vi "Configure Digital Channel.vi"(5 "Threshold (1.4 V)":dbl=1.4, 6 "Channel Size (1: Medium)":i32(ring)=1 items=["Small", "Medium", "Large"], 7 "Channel Position (0)":dbl, 8 "error in (no error)":errorcluster, 9 "Enable Display (F: Disable)":bool, 10 "Channel Name (0: D0)":i32(ring) items=["D0", "D1", "D2", "D3", "D4", "D5", "D6", "D7", "D8", "D9", "D10", "D11", "D12", "D13", "D14", "D15"], 11 "VISA resource name":refnum<visa-resource-name>) -> (0 "error out":errorcluster, 3 "VISA resource name out":refnum<visa-resource-name>)   [LabVIEW 2015, in "Agilent 2000 3000 X-Series.lvlib"]
doc: "Configures the digital channel.\n\n<B>Note(s):</B>\nThis function is only applicable for MSO models."
uses:
  Agilent 2000 3000 X-Series.lvlib
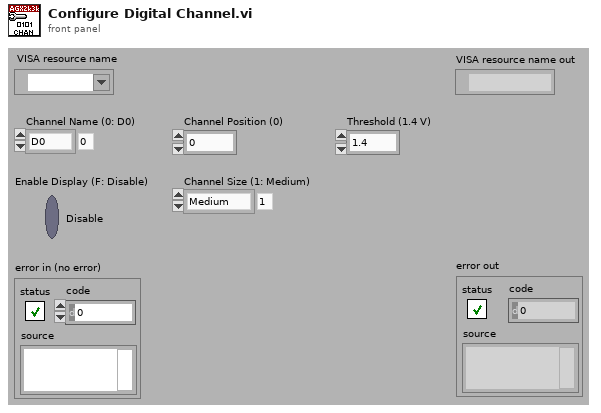
[diagram p1: front panel]
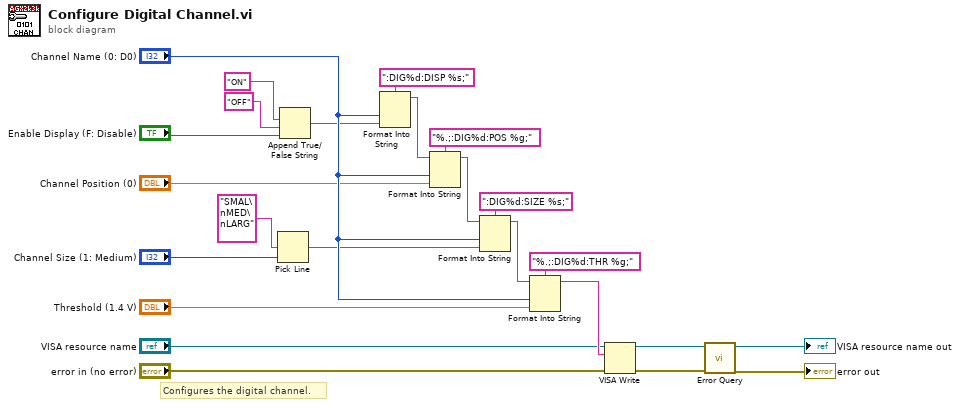
[diagram p0: block diagram]
diagram:
  # "Configures the digital channel."
  n1 = Pick Line(multi-line string="SMAL\nMED\nLARG", line index="Channel Size (1: Medium)") -> (output string=w11:string)  [unwired: 1 out]
  n2 = Append True/False String(1:"Enable Display (F: Disable)", 2:"OFF", 3:"ON") -> (0:w19:string)  [unwired: 1 out]
  n3 = Format Into String(format string=":DIG%d:DISP %s;", "Channel Name (0: D0)", w19) -> (resulting string=w18:string)  [unwired: 2 in, 1 out]
  n4 = Format Into String(format string="%.;:DIG%d:POS %g;", initial string=w18, "Channel Name (0: D0)", "Channel Position (0)") -> (resulting string=w13:string)  [unwired: 1 in, 1 out]
  n5 = Format Into String(format string=":DIG%d:SIZE %s;", initial string=w13, "Channel Name (0: D0)", w11) -> (resulting string=w10:string)  [unwired: 1 in, 1 out]
  n6 = Format Into String(format string="%.;:DIG%d:THR %g;", initial string=w10, "Channel Name (0: D0)", "Threshold (1.4 V)") -> (resulting string=w7:string)  [unwired: 1 in, 1 out]
  n7 = VISA Write(VISA resource name="VISA resource name", write buffer=w7, error in (no error)="error in (no error)") -> (VISA resource name out=w4:refnum<visa-resource-name>, error out=w3:errorcluster)  [unwired: 1 out]
  n8 = call "Error Query.vi"("error in (no error)"=w3, "VISA resource name"=w4) -> ("error out"=→"error out":errorcluster, "VISA resource name out"=→"VISA resource name out":refnum<visa-resource-name>)  [unwired: 8 out]
